vi "Get UUID.vi"(8 "error in (no error)":errorcluster, 11 "Output in":refnum<class "Output.lvclass">) -> (0 "error out":errorcluster, 2 "UUID":string, 3 "Output out":refnum<class "Output.lvclass">)   [LabVIEW 2015, in "Output.lvclass"]
uses:
  Output.lvclass
  Output.lvclass/Output.ctl
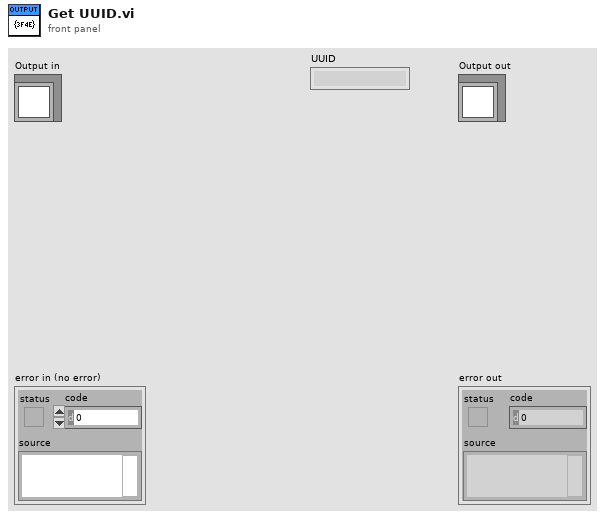
[diagram p1: front panel]
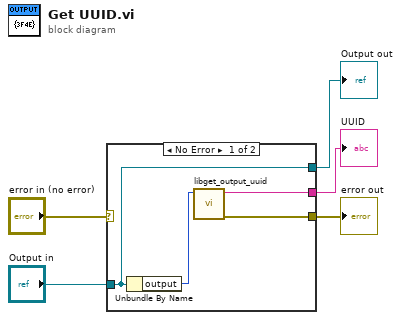
[diagram p0: block diagram]
diagram:
  n1 = case shown="No Error" "error in (no error)" {
    selector: "error in (no error)" -> [_ w11]
    tunnel: [w6 w11] -> w4
    tunnel: [w9 w10] -> w2
    tunnel: "Output in" -> [w9 w10]
    tunnel: [w7 _] -> w1
    frame No Error {
      n2 = Unbundle By Name(w9) -> ("output"=w8:i32)
      n3 = call "libget_output_uuid.vi"("output"=w8) -> ("error out"=w6:errorcluster, "UUID"=w7:string)  [unwired: 9 in]
    }
    frame Error {
    }
  }
  "error out" <- w4
  "Output out" <- w2
  "UUID" <- w1
